vi "ini.vi"(8 "error in (no error)":errorcluster, 11 "Caculator in":refnum<class "Caculator.lvclass">) -> (0 "error out":errorcluster, 3 "Caculator out":refnum<class "Caculator.lvclass">)   [LabVIEW 2017, in "Caculator.lvclass"]
uses:
  Caculator.lvclass
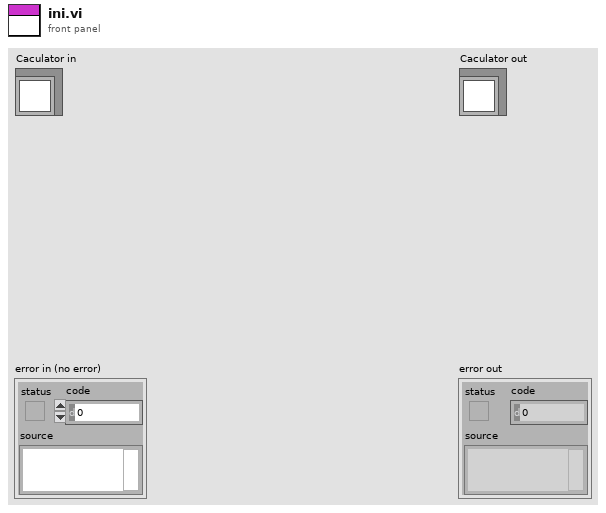
[diagram p1: front panel]
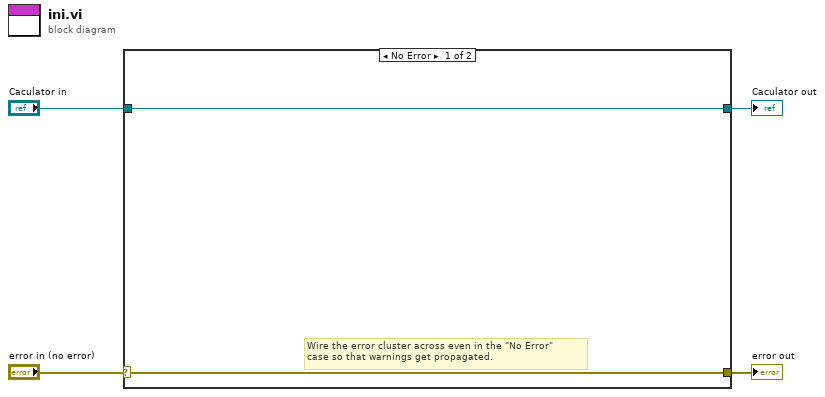
[diagram p0: block diagram]
diagram:
  n1 = case shown="No Error" "error in (no error)" {
    selector: "error in (no error)" -> [w6 w8]
    tunnel: [w6 w8] -> w3
    tunnel: [w5 w7] -> w1
    tunnel: "Caculator in" -> [w5 w7]
    frame No Error {
      # "Wire the error cluster across even in the \"No Error\"\ncase so that warnings get propagated."
    }
    frame Error {
    }
  }
  "error out" <- w3
  "Caculator out" <- w1
